vi "Live Display and capture_2.vi"() -> ()   [LabVIEW 2020]
doc: "The Acquire Every Image (Optimized Performance) example shows the basics of using a ring acquisition. There are some camera restrictions to using this mode that are described in more detail in the block diagram of the VI, but it is recommended to use this method for performance-critical applications when possible."
uses:
  <vilib>/vision/driver/NI_Vision_Acquisition_Software.lvlib
  <vilib>/vision/driver/IMAQdx.llb/IMAQdx Buffer Number Mode.ctl
  <vilib>/vision/driver/IMAQdx.llb/IMAQdx Acquisition Mode.ctl
  <resource>/objmgr/imaqdx.rc
  Camera Server/Globals/CamServer global.vi
  <vilib>/userDefined/High Color/IMAQdx.ctl
panel:
  out "Array":T1[](array[typedef])
  out "Name 2":string
  out "Name 1":string
  out "Image 2":T2(plugin-control)
  out "error out":errorcluster
  out "Image count":i32
  out "Image 1":T2(plugin-control)
  in  "Stop":bool
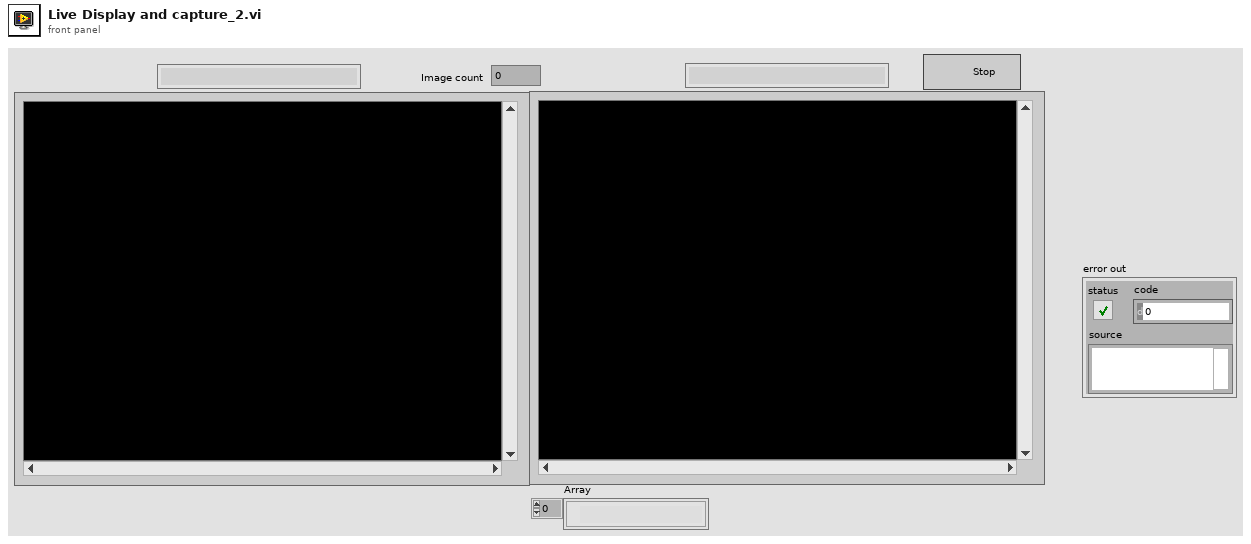
[diagram p1: front panel]
types:
  T1 = typedef "IMAQdx.ctl" = refnum<k21>
  T2 = typedef "IMAQ Image.ctl" = refnum<image>
  T3 = typedef "NI_Vision_Acquisition_Software.lvlib/IMAQdx Acquisition Mode.ctl" = enum32{"One Shot", "Continuous"}
  T4 = typedef "NI_Vision_Acquisition_Software.lvlib/IMAQdx Buffer Number Mode.ctl" = enum32{"Next", "Last", "Buffer Number", "Every", "Last New"}
  T5 = typedef "Camera enum.ctl" = string
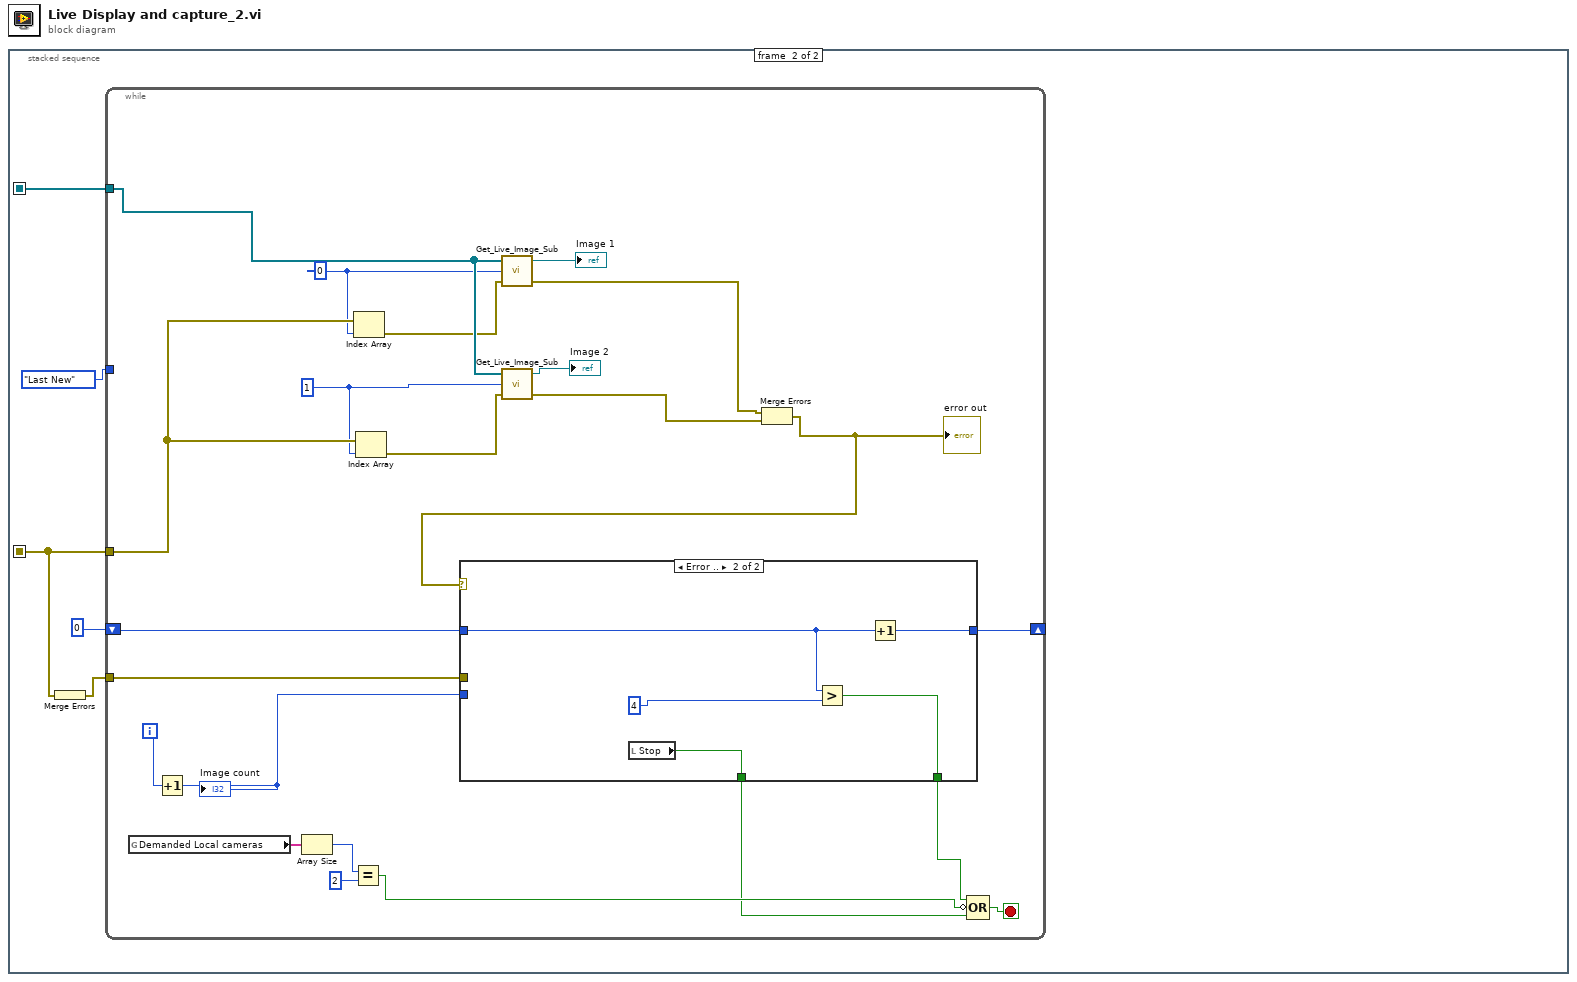
[diagram p0: block diagram]
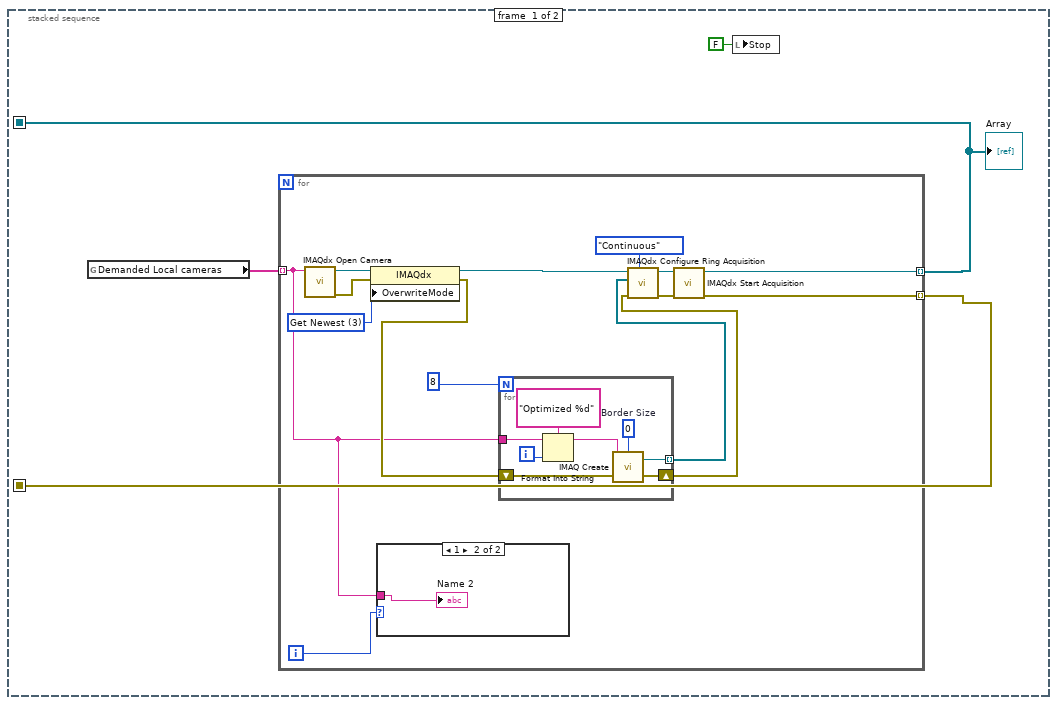
[diagram p2: hidden frame]
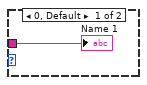
[diagram p3: hidden frame]
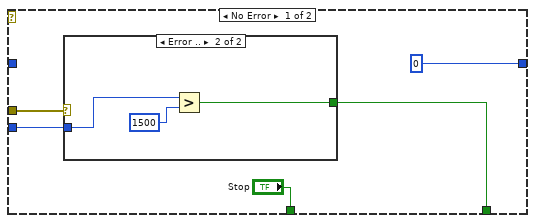
[diagram p4: hidden frame]
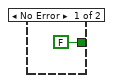
[diagram p5: hidden frame]
diagram:
  n1 = stacked-sequence {
    seq-local: [w4 _] -> [_ w34]
    seq-local: [w3 _] -> [_ w31]
    frame #0 {
      n2 = global read "CamServer global.vi" "Demanded Local cameras"() -> (w2:T5[])
      n3 = for {
        tunnel: w2 -> [w5] mode=indexing
        tunnel: [w13] -> w4 mode=indexing
        tunnel: [w12] -> w3 mode=indexing
        i -> [w6]
        w7 = u32 3 items=["Get Oldest"=0, "Fail"=2, "Get Newest"=3] ("OverwriteMode")
        n4 = call <vilib>:"IMAQdx Open Camera.vi"("Session In"=w5) -> ("error out"=w19:errorcluster, "Session Out"=w18:T1)  [unwired: 2 in, 7 out]
        n5 = property class="IMAQdx"(reference=w18, error in=w19, "OverwriteMode"=w7) -> (reference out=w14:T1, error out=w11:errorcluster)
        n6 = case shown="1" w6 {
          tunnel: w5 -> [w20 w21]
          frame 0, Default {
            "Name 1" <- w20
          }
          frame 1 {
            "Name 2" <- w21
          }
        }
        n7 = for {
          N: 8 ("Number of Images") -> [_]
          tunnel: [w28] -> w9 mode=indexing
          shift-right: [w27] -> w10
          shift-left: w11 -> [w29]
          tunnel: w5 -> [w22]
          i -> [w26]
          w23 = 0  # Border Size
          n8 = Format Into String(format string="Optimized %d" ("Image Name"), initial string=w22, w26) -> (resulting string=w25:string)  [unwired: 1 in, 1 out]
          n9 = call "IMAQ Create"("Border Size"=w23, "Image Name"=w25, "error in (no error)"=w29) -> ("New Image"=w28:T2, "error out"=w27:errorcluster)  [unwired: 1 in, 1 out]
        }
        n10 = call <vilib>:"IMAQdx Configure Ring Acquisition.vi"("Mode"=IMAQdx_Acquisition_Mode."Continuous" ("Continuous?"), "error in"=w10, "Images"=w9, "Session In"=w14) -> ("error out"=w16:errorcluster, "Session Out"=w15:T1)  [unwired: 5 in, 1 out]
        n11 = call <vilib>:"IMAQdx Start Acquisition.vi"("error in"=w16, "Session In"=w15) -> ("error out"=w12:errorcluster, "Session Out"=w13:T1)  [unwired: 8 out]
      }
      "Array" <- w4
      n12 = local write "Stop"(FALSE ("Stop")) -> ()
    }
    frame #1 {
      n13 = Merge Errors(w31) -> (w30:errorcluster)
      n14 = while {
        tunnel: w34 -> [w47]
        tunnel: w31 -> [w43]
        tunnel: IMAQdx_Buffer_Number_Mode."Last New" ("Buffer Number Mode") -> [_]
        shift-right: [w46] -> _
        shift-left: 0 -> [w45]
        tunnel: w30 -> [w38]
        i -> [w52]
        stop <- w57 stop-if-true
        w40 = 1 ("y")
        w42 = 0 ("y")
        n15 = global read "CamServer global.vi" "Demanded Local cameras"() -> (w56:T5[])
        n16 = Increment(x=w52) -> (x+1=w37:i32)
        "Image count" <- w37
        n17 = Array Size(array=w56) -> (size(s)=w55:i32)
        n18 = Equal?(x=w55, y=2) -> (x = y?=w54:bool)
        n19 = Index Array(array=w43, index=w42) -> (element=w41:errorcluster)
        n20 = Index Array(array=w43, index=w40) -> (element=w39:errorcluster)
        n21 = call "Get_Live_Image_Sub.vi"("error in"=w41, "index"=w42, "Session Array"=w47) -> ("error out"=w50:errorcluster, "Image"=→"Image 1":T2)  [unwired: 1 in]
        n22 = call "Get_Live_Image_Sub.vi"("error in"=w39, "index"=w40, "Session Array"=w47) -> ("error out"=w48:errorcluster, "Image"=→"Image 2":T2)  [unwired: 1 in]
        n23 = Merge Errors(w50, w48) -> (w35:errorcluster)
        "error out" <- w35
        n24 = case shown="Error .." w35 {
          tunnel: [0 w71] -> w46
          tunnel: w45 -> [_ w70]
          tunnel: [w59 w69] -> w36
          tunnel: w38 -> [w61 _]
          tunnel: w37 -> [w60 _]
          tunnel: ["Stop" w67] -> w44
          frame No Error {
            n25 = case shown="Error .." w61 {
              tunnel: w60 -> [_ w65]
              tunnel: [FALSE w64] -> w59
              frame No Error {
              }
              frame Error {
                n26 = Greater?(x=w65, y=1500) -> (0:w64:bool)
              }
            }
          }
          frame Error {
            n27 = local read "Stop"() -> (w67:bool)
            n28 = Greater?(x=w70, y=4) -> (0:w69:bool)
            n29 = Increment(x=w70) -> (x+1=w71:i32)
          }
        }
        n30 = Compound Arithmetic op=OR(w36, invert w54, w44) -> (w57:bool)
      }
    }
  }
